vi "Test Decode JSON.vi"(8 "error in (no error)":errorcluster) -> (0 "error out":errorcluster)   [LabVIEW 2019]
uses:
  f8c5686a-5e9b-4782-9975-992b5e36aacc.vi
  f8c5686a-5e9b-4782-9975-992b5e36aacc.vi/ea02b668-b91e-429e-b720-e502299c0107.vi
  f8c5686a-5e9b-4782-9975-992b5e36aacc.vi/50262bde-9363-47c6-8c17-5d5d26c9cd6d.vi
  <vilib>/Utility/Data Type/Get Type Information.vi
  <vilib>/JDP Science/JSONtext/JSON text to Variant.vi
  <vilib>/JDP Science/JSONtext/LVClass Serializer/JSONtext LVClass Serializer.lvclass
  JSON-RPC/JSON-RPC/JSON-RPC.lvclass
  <vilib>/addons/_JKI Toolkits/Caraya/classes/Assert/Assert.lvclass
  <vilib>/addons/_JKI Toolkits/Caraya/classes/Test/Test.lvclass
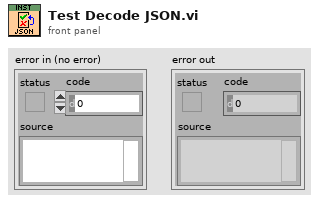
[diagram p1: front panel]
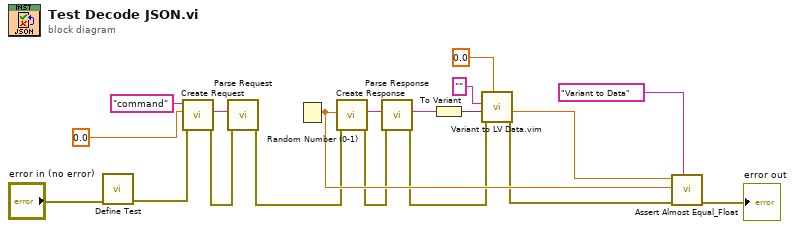
[diagram p0: block diagram]
diagram:
  n1 = call <vilib>:"Define Test.vi"("error in (no error)"="error in (no error)") -> ("error out"=w4:errorcluster)  [unwired: 10 in]
  n2 = call "Create Request.vi"("error in (no error)"=w4, "params"=0.0, "method"="command") -> ("error out"=w6:errorcluster, "{JSON} Requests"=w18:string)  [unwired: 5 in, 2 out]
  n3 = call "Parse Request.vi"("error in (no error)"=w6, "{JSON} Request"=w18) -> ("error out"=w7:errorcluster)  [unwired: 5 in, 4 out]
  n4 = Random Number (0-1)() -> (number: 0 to 1=w11:dbl)
  n5 = call "Create Response.vi"("error in (no error)"=w7, "result"=w11) -> ("error out"=w8:errorcluster, "{JSON} Response"=w16:string)  [unwired: 7 in, 1 out]
  n6 = call "Parse Response.vi"("error in (no error)"=w8, "{JSON} Response"=w16) -> ("error out"=w9:errorcluster, "results"=w15:string)  [unwired: 5 in, 3 out]
  n7 = To Variant(anything=w15) -> (Variant=w14:variant)
  n8 = call "Variant to LV Data.vim"("type"=0.0, "error in (no error)"=w9, "JSON Data in"=w14, "Command"="") -> ("error out"=w5:errorcluster, "Data out"=w13:dbl)  [unwired: 4 in, 2 out]
  n9 = call <vilib>:"Assert Almost Equal_Float.vi"("Label"="Variant to Data", "error in (no error)"=w5, "Y"=w11, "X"=w13) -> ("error out"=→"error out":errorcluster)  [unwired: 7 in]
